vi "Create ByteFIFO.vi"(7 "Allow Overflow? (T)":bool=TRUE, 8 "error in":errorcluster, 10 "default value":u8 format="%02x", 11 "bufSize":i32) -> (0 "error out":errorcluster, 3 "Buffer":refnum<data-value>)   [LabVIEW 2013, in "CircularBuffer.lvlib" / "ByteFIFO.lvclass"]
doc: "This VI creates a ring buffer of set size. This buffer is created in one place in the memory and is then accessed via pointer/reference.\n\nThe Data Type input is required because it defines the place in the memory to correct size thus removing the need for memory reallocation."
uses:
  ByteFIFO.lvclass
  VariantBuffer/buffer-type -- enum.ctl
  VariantBuffer/VariantBuffer.lvclass
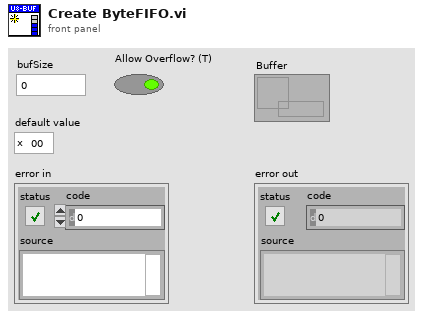
[diagram p1: front panel]
types:
  T1 = typedef "CircularBuffer.lvlib/VariantBuffer.lvclass/buffer-type -- enum.ctl" = enum16{"Queue", "Stack"}
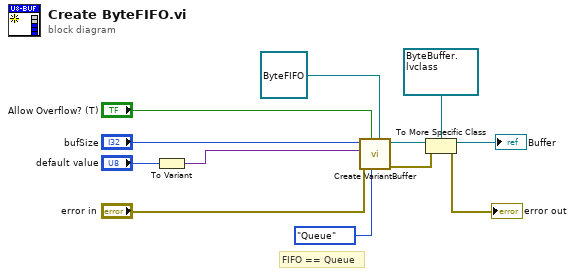
[diagram p0: block diagram]
diagram:
  # "FIFO == Queue"
  n1 = To Variant(anything="default value") -> (Variant=w9:variant)
  n2 = call "Create VariantBuffer.vi"("Buffer"=refnum<class "ByteFIFO.lvclass"> refnum ("ByteBuffer.lvclass"), "buffer-type"=buffer-type_--_enum."Queue", "Allow Overflow? (T)"="Allow Overflow? (T)", "error in"="error in", "default"=w9, "bufSize"="bufSize") -> ("error out"=w4:errorcluster, "Buffer"=w7:refnum<data-value>)  [unwired: 4 in]
  n3 = To More Specific Class(target class=refnum<data-value> refnum ("Buffer"), reference=w7, error in=w4) -> (specific class reference=→"Buffer":refnum<data-value>, error out=→"error out":errorcluster)
